vi "Menu Resolve Source Str.vi"(0 "字符串":string) -> (1 "菜单信息":cluster{"父菜单名":string, "菜单项":string[]}[](array[cluster]), 2 "菜单详情":T2(array[cluster]))   [LabVIEW 2011]
uses:
  <vilib>/Utility/miscctls.llb/LVMenuShortCut.ctl
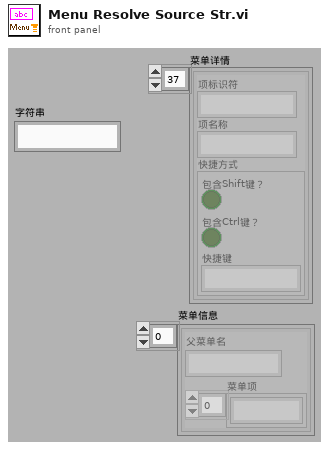
[diagram p1: front panel]
types:
  T1 = typedef "LVMenuShortCut.ctl" = cluster{"Include Shift Key?":bool, "Include Ctrl Key?":bool, "Shortcut Key":string}
  T2 = cluster{"项标识符":string, "项名称":string, "快捷方式":T1}[]
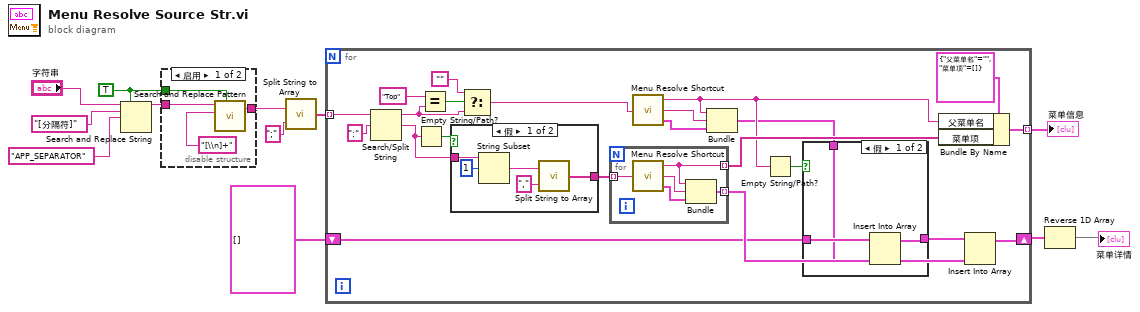
[diagram p0: block diagram]
diagram:
  w2 = TRUE ("替换全部？(F)")
  n1 = Search and Replace String(replace all?=w2, input string="字符串", search string="[分隔符]" ("搜索字符串"), replace string="APP_SEPARATOR" ("替换字符串(\"\")")) -> (result string=w3:string)  [unwired: 1 in, 6 out]
  n2 = disable-structure shown="启用" {
    disable-tunnel: w3 -> [w16 w17]
    disable-tunnel: w2 -> [w15 _]
    disable-tunnel: [w14 w17] -> w1
    frame Enabled {
      n3 = call <vilib>:"Search and Replace Pattern.vi"("string"=w16, "regular expression (\"\")"="[\\n]+" ("regular expression (\"\")"), "replace all? (F)"=w15) -> ("result string"=w14:string)  [unwired: 2 in, 1 out]
    }
    frame Disabled {
    }
  }
  n4 = call "Split String to Array.vi"("搜索字符串/字符(-)"=";", "字符串"=w1) -> ("字符串数组"=w12:string[])
  n5 = for {
    tunnel: w12 -> [w39] mode=indexing
    tunnel: [w30] -> w11 mode=indexing
    shift-right: [w18] -> w5
    shift-left: T2 [] -> [w20]
    n6 = Search/Split String(string=w39, search string/char (-)=":" ("搜索字符串/字符(-)")) -> (substring before match=w35:string, match + rest of string=w32:string)  [unwired: 2 out]
    n7 = Empty String/Path?(string/path=w32) -> (empty?=w33:bool)
    n8 = Equal?(x="Top", y=w35) -> (x = y?=w36:bool)
    n9 = case shown="假" w33 {
      tunnel: w32 -> [w53 _]
      tunnel: [w49 _] -> w28
      frame False {
        n10 = String Subset(string=w53, offset (0)=1 ("偏移量(0)")) -> (substring=w51:string)  [unwired: 1 out]
        n11 = call "Split String to Array.vi"("搜索字符串/字符(-)"=",", "字符串"=w51) -> ("字符串数组"=w49:string[])
      }
      frame True {
      }
    }
    n12 = Select(t="", s=w36, f=w35) -> (s? t:f=w29:string)
    n13 = for {
      tunnel: w28 -> [w48] mode=indexing
      tunnel: [w47] -> w27 mode=indexing
      tunnel: [w44] -> w21 mode=indexing
      n14 = call "Menu Resolve Shortcut.vi"("输入字符串"=w48) -> ("快捷方式"=w45:T1, "项名称"=w46:string, "项标识符"=w47:string)
      n15 = Bundle("项标识符"=w47, "项名称"=w46, "快捷方式"=w45) -> (w44:cluster{"项标识符":string, "项名称":string, "快捷方式":T1})  [unwired: 1 in]
    }
    n16 = call "Menu Resolve Shortcut.vi"("输入字符串"=w29) -> ("快捷方式"=w23:T1, "项名称"=w24:string, "项标识符"=w25:string)
    n17 = Bundle("项标识符"=w25, "项名称"=w24, "快捷方式"=w23) -> (w22:cluster{"项标识符":string, "项名称":string, "快捷方式":T1})  [unwired: 1 in]
    n18 = Empty String/Path?(string/path=w25) -> (empty?=w26:bool)
    n19 = case shown="假" w26 {
      tunnel: w22 -> [w41 _]
      tunnel: w20 -> [w42 w43]
      tunnel: [w40 w43] -> w19
      frame False {
        n20 = Insert Into Array(array=w42, new element=w41) -> (w40:T2)  [unwired: 1 in]
      }
      frame True {
      }
    }
    n21 = Bundle By Name(cluster=cluster{"父菜单名":string, "菜单项":string[]} {"父菜单名"="", "菜单项"=[]} ("菜单项"), "父菜单名"=w25, "菜单项"=w27) -> (w30:cluster{"父菜单名":string, "菜单项":string[]})
    n22 = Insert Into Array(array=w19, new element=w21) -> (w18:T2)  [unwired: 1 in]
  }
  "菜单信息" <- w11
  n23 = Reverse 1D Array(array=w5) -> (reversed array=→"菜单详情":T2)
